vi "Read position.vi"(8 "error in (no error)":errorcluster, 11 "KST101 in":refnum<class "KST101.lvclass">) -> (0 "error out":errorcluster, 2 "position":dbl, 3 "KST101 out":refnum<class "KST101.lvclass">)   [LabVIEW 2016, in "Stepper Motor Controller.lvlib" / "KST101.lvclass"]
uses:
  KST101.lvclass
  KST101.lvclass/KST101.ctl
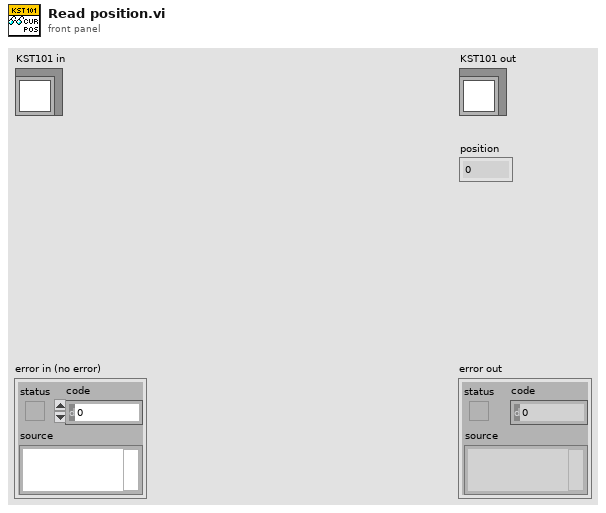
[diagram p1: front panel]
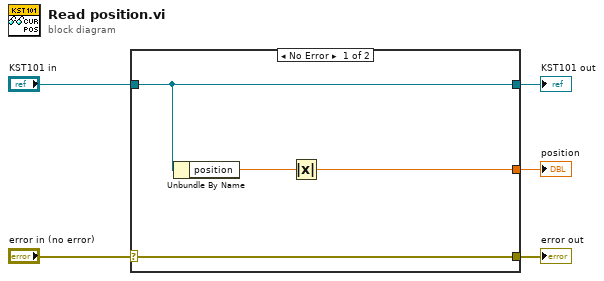
[diagram p0: block diagram]
diagram:
  n1 = case shown="No Error" "error in (no error)" {
    selector: "error in (no error)" -> [w9 w10]
    tunnel: [w9 w10] -> w4
    tunnel: [w8 w11] -> w2
    tunnel: "KST101 in" -> [w8 w11]
    tunnel: [w6 _] -> w1
    frame No Error {
      n2 = Unbundle By Name(w8) -> ("position"=w7:dbl)
      n3 = Absolute Value(x=w7) -> (abs(x)=w6:dbl)
    }
    frame Error {
    }
  }
  "error out" <- w4
  "KST101 out" <- w2
  "position" <- w1
